vi "Main.vi"(10 "COM port name":refnum<visa-resource-name>, 11 "Module Admin":refnum<class "Delacor_lib_QMH_Cloneable Module Admin.lvclass">) -> ()   [LabVIEW 2018, in "CE14_v2.lvlib"]
doc: "This template is based off of the Queued Message Handler design pattern and the Queued Message Handler project template that ships with LabVIEW.\n\nThe main difference is that the queue is private to this module and communication between modules is performed via Broadcast and Request events.\n\nRequest events are wrapped in public API methods and are handled in the Event Handling Loop (EHL) of this VI. Any module can register for Broadcast events sent by this module. The EHL generates messages based on user interface actions.\n\nThe Message Handling Loop (MHL) processes messages generated by the EHL, or by other messages. The messages are string values, so new messages can be added easily to the Message Cases case structure in the MHL. Each message cluster can also provide an optional value for Message Data, which is a variant that can be converted to whatever message-specific data is required.\n_____\nBased on DQMH Project Template 6.0.0.91."
uses:
  CE14_v2.lvlib
  <vilib>/Delacor/Delacor QMH/Libraries/Cloneable Module Admin_class/Delacor_lib_QMH_Cloneable Module Admin.lvclass
  C:/Program Files (x86)/National Instruments/LabVIEW 2018/vi.lib/Delacor/Delacor QMH/Libraries/Module Admin_class/Delacor_lib_QMH_Module Admin.lvclass
  <vilib>/Delacor/Delacor QMH/Libraries/Message Queue_class/Delacor_lib_QMH_Message Queue.lvclass/Delacor_lib_QMH_Message Queue.ctl
  Module Data--cluster.ctl
  <vilib>/Delacor/Delacor QMH/Libraries/Cloneable Module Admin_class/Delacor_lib_QMH_Cloneable Module Admin.lvclass/Delacor_lib_QMH_Cloneable Module Admin.ctl
  Stop Argument--cluster.ctl
  <vilib>/Delacor/Delacor QMH/Libraries/Module Admin_class/Delacor_lib_QMH_Module Admin.lvclass/Delacor_lib_QMH_Module Admin.ctl
  CE14.CheckConnected Argument--cluster.ctl
  CE14.CheckConnected (Reply Payload)--cluster.ctl
  Read AC parameters Argument--cluster.ctl
  Connect to CE14 Argument--cluster.ctl
  <vilib>/Utility/miscctls.llb/LVPointTypeDef.ctl
  <vilib>/Delacor/Delacor QMH/Libraries/Message Queue_class/Delacor_lib_QMH_Enqueue Message (Single).vi
  <vilib>/Delacor/Delacor QMH/Libraries/Cloneable Module Admin_class/Delacor_lib_QMH_Get Module ID.vi
  <vilib>/Delacor/Delacor QMH/Libraries/Module Admin_class/Delacor_lib_QMH_Get External Launch.vi
  <vilib>/Utility/error.llb/Error Cluster From Error Code.vi
  <vilib>/ErrorRing/Error Ring.xnode
  <vilib>/Delacor/Delacor QMH/Libraries/Message Queue_class/Delacor_lib_QMH_Message Queue.lvclass
  Instrument Drivers/LVdriver_CE14(eMIC)/CE14_eMIC.lvlib
panel:
  out "Frequency":dbl
  out "connected":bool
  out "error out":errorcluster
  out "Status":string
  in  "Simulate EHL Error":bool
  in  "Simulate MHL Error":bool
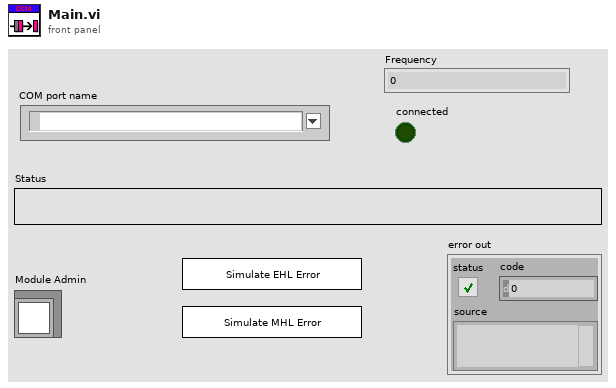
[diagram p1: front panel]
types:
  T1 = typedef "CE14_v2.lvlib/Request Events--cluster.ctl" = cluster{"Stop Module":refnum<user-event>, "Show Panel":refnum<user-event>, "Hide Panel":refnum<user-event>, "Show Diagram":refnum<user-event>, "Get Module Execution Status":refnum<user-event>, "CE14.CheckConnected":refnum<user-event>, "Read AC parameters":refnum<user-event>, "Connect to CE14":refnum<user-event>, "Stop helper loop":refnum<user-event>, "Start Helper Loop":refnum<user-event>}
  T2 = typedef "CE14_v2.lvlib/Module Data--cluster.ctl" = cluster{"Status":string, "VISA resource name":refnum<visa-resource-name>, "connected":bool}
  T3 = enum32{"invalid lock state", "Not Locked", "Locked (No Password)", "Password-protected"}
  T4 = typedef "CE14_v2.lvlib/Stop Argument--cluster.ctl" = cluster{"Module ID":i32, "Origin":string, "Exit via Stop Module Req?":bool, "Wait for Module to stop?":bool}
  T5 = typedef "CE14_v2.lvlib/CE14.CheckConnected Argument--cluster.ctl" = cluster{"Module ID":i32, "Wait Notifier":refnum<notifier>, "wait for reply":bool}
  T6 = typedef "CE14_v2.lvlib/Read AC parameters Argument--cluster.ctl" = cluster{"Module ID":i32, "Boolean":bool}
  T7 = typedef "CE14_v2.lvlib/Connect to CE14 Argument--cluster.ctl" = cluster{"Module ID":i32, "Boolean":bool}
  T8 = typedef "LVPointTypeDef.ctl" = cluster{"Horizontal":i16, "Vertical":i16}
  T9 = enum32{"Invalid", "Standard", "Closed", "Hidden", "Minimized", "Maximized"}
  T10 = typedef "CE14_v2.lvlib/CE14.CheckConnected (Reply Payload)--cluster.ctl" = cluster{"Success":bool, "CE14.CheckConnected_error":errorcluster}
  T11 = typedef "CE14_eMIC.lvlib/CE14.data.ctl" = cluster{"string":string, "float":dbl, "Name":string}
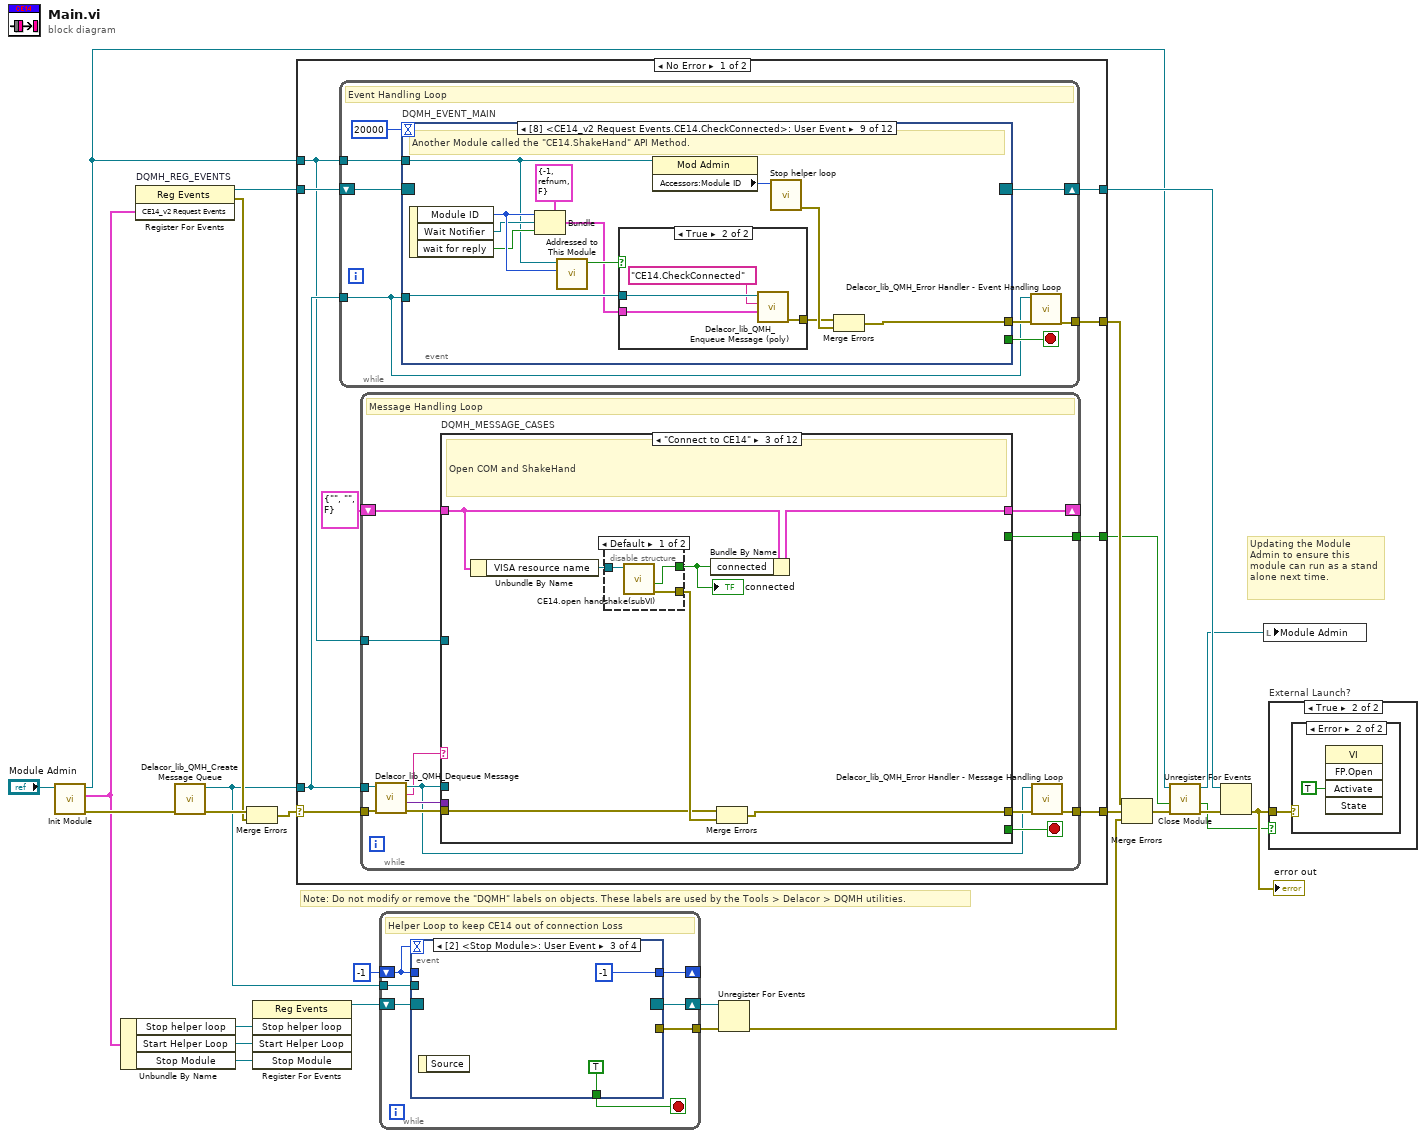
[diagram p0: block diagram]
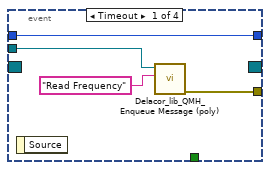
[diagram p2: hidden frame]
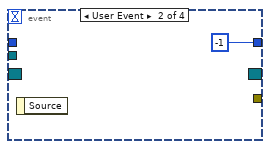
[diagram p3: hidden frame]
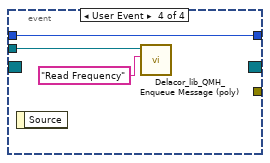
[diagram p4: hidden frame]
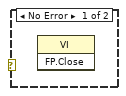
[diagram p6: hidden frame]
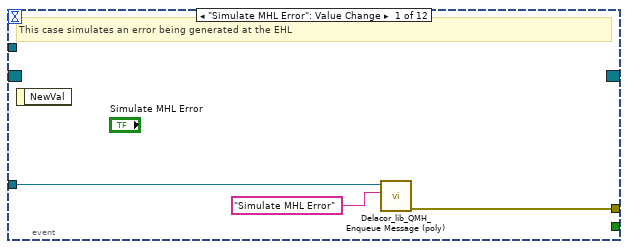
[diagram p7: hidden frame]
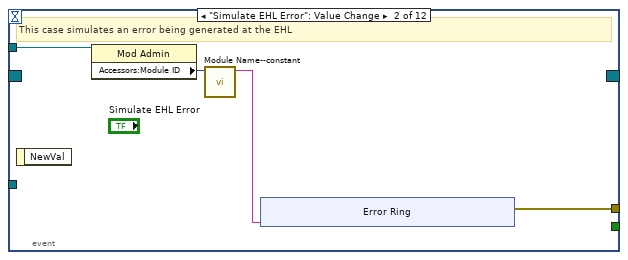
[diagram p8: hidden frame]
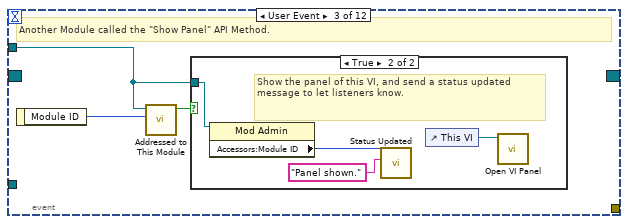
[diagram p9: hidden frame]
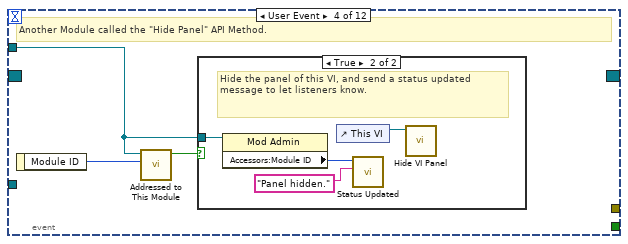
[diagram p11: hidden frame]
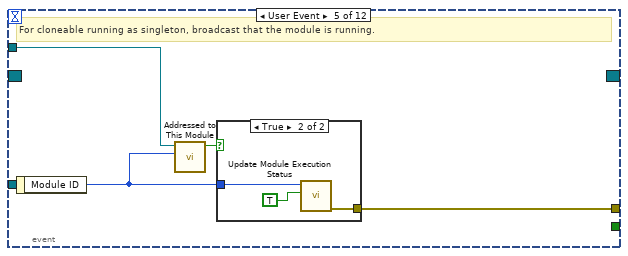
[diagram p13: hidden frame]
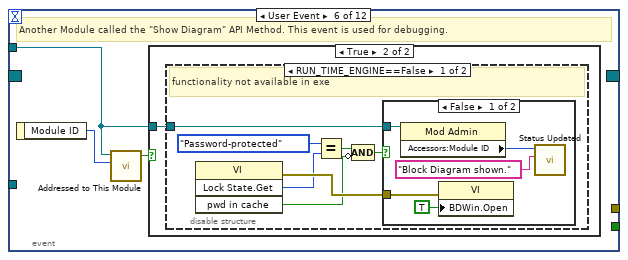
[diagram p15: hidden frame]
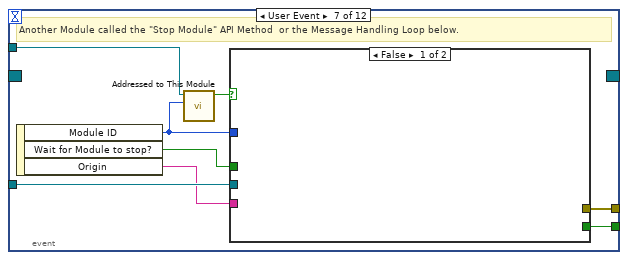
[diagram p19: hidden frame]
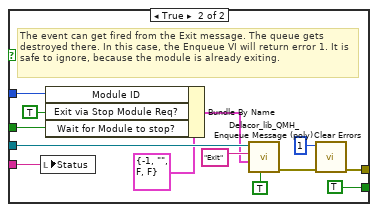
[diagram p20: hidden frame]
diagram:
  # "Note: Do not modify or remove the \"DQMH\" labels on objects. These labels are used by the Tools > Delacor > DQMH utilities."
  # "Updating the Module Admin to ensure this module can run as a stand alone next time."
  n1 = call "Init Module.vi"("Cloneable Module Admin in"="Module Admin") -> ("error out"=w23:errorcluster, "CE14_v2 Request Events"=w9:T1, "Cloneable Module Admin out"=w15:refnum<class "Delacor_lib_QMH_Cloneable Module Admin.lvclass">)  [unwired: 8 in]
  n2 = Unbundle By Name(w9) -> ("Stop helper loop"=w6:refnum<user-event>, "Start Helper Loop"=w5:refnum<user-event>, "Stop Module"=w4:refnum<user-event>)
  n3 = register-events "DQMH_REG_EVENTS"(w9) -> (reference out=w11:refnum<event-registration>, error out=w18:errorcluster)  [unwired: 2 in]
  n4 = call <vilib>:"Delacor_lib_QMH_Create Message Queue.vi"("error in"=w23) -> ("error out"=w20:errorcluster, "Message Queue"=w10:refnum<class "Delacor_lib_QMH_Message Queue.lvclass">)  [unwired: 9 in]
  n5 = Merge Errors(w20, w18) -> (w19:errorcluster)
  n6 = register-events(w6, w5, w4) -> (reference out=w8:refnum<event-registration>)  [unwired: 2 in, 1 out]
  n7 = case shown="No Error" w19 {
    selector: w19 -> [w33 w349]
    tunnel: [w35 w348] -> w24
    tunnel: [w32 w356] -> w17
    tunnel: w11 -> [w30 w356]
    tunnel: w10 -> [w29 w347]
    tunnel: [w34 _] -> w25
    tunnel: w15 -> [w28 w352]
    tunnel: [w27 _] -> w13
    frame No Error {
      n8 = while {
        tunnel: w29 -> [w37]
        shift-right: [w40] -> w32
        shift-left: w30 -> [w41]
        tunnel: [w42] -> w34
        tunnel: w28 -> [w38]
        stop <- w39 stop-if-true
        # "Event Handling Loop"
        n9 = event "DQMH_EVENT_MAIN" shown="[8] <CE14_v2 Request Events.CE14.CheckConnected>: User Event" {
          selector: w41 -> [_ _ _ _ _ _ _ _ _ _ _ _]
          dyn-events: [_ _ _ _ _ _ _ _ _ _ _ _] -> w40
          timeout: 20000 -> [_ _ _ _ _ _ _ _ _ _ _ _]
          tunnel: [_ _ _ _ _ _ w99 _ _ _ _ _] -> w39
          tunnel: w37 -> [w45 _ _ _ _ _ w101 w117 w137 w152 w167 _]
          tunnel: [w46 w50 _ _ w75 _ w102 w120 w127 w142 w158 _] -> w43
          tunnel: w38 -> [_ w49 w58 w65 w73 w79 w95 w118 w126 w145 w159 w172]
          event "Simulate MHL Error": Value Change {
            # "This case simulates an error being generated at the EHL"
            n10 = event-data() -> ()  [unwired: 1 in, 1 out]
            n11 = call-poly <vilib>:"Delacor_lib_QMH_Enqueue Message (poly).vi"("Message"="Simulate MHL Error", "Message Queue in"=w45) -> ("error out"=w46:errorcluster)  [unwired: 8 in, 1 out]
          }
          event "Simulate EHL Error": Value Change {
            # "This case simulates an error being generated at the EHL"
            n12 = event-data() -> ()  [unwired: 1 in, 1 out]
            n13 = property class="Mod Admin"(reference=w49) -> ("Accessors:Module ID"=w48:i32)  [unwired: 1 in, 2 out]
            n14 = call "Module Name--constant.vi"("Module ID"=w48) -> ("Module Name"=w47:string)  [unwired: 10 in]
            n15 = xnode "Error Ring"("parameter 0"=w47) -> ("error out"=w50:errorcluster)
          }
          event User Event {
            # "Another Module called the \"Show Panel\" API Method."
            n16 = event-data() -> ("Module ID"=w59:i32)  [unwired: 1 in]
            n17 = call "Addressed to This Module.vi"("Module ID from Argument"=w59, "Module Admin"=w58) -> ("Addressed to this instance?"=w60:bool)  [unwired: 8 in, 1 out]
            n18 = case shown="True" w60 {
              tunnel: w58 -> [_ w62]
              frame False {
              }
              frame True {
                # "Show the panel of this VI, and send a status updated message to let listeners know."
                n19 = property class="Mod Admin"(reference=w62) -> ("Accessors:Module ID"=w61:i32)  [unwired: 1 in, 2 out]
                n20 = call "Status Updated.vi"("Status"="Panel shown." ("format string"), "Module ID"=w61) -> ()  [unwired: 9 in, 1 out]
                n21 = control-ref of="This VI"() -> (w64:refnum<vi>)
                n22 = call "Open VI Panel.vi"("VI"=w64) -> ()  [unwired: 10 in, 1 out]
              }
            }
          }
          event User Event {
            # "Another Module called the \"Hide Panel\" API Method."
            n23 = event-data() -> ("Module ID"=w66:i32)  [unwired: 1 in]
            n24 = call "Addressed to This Module.vi"("Module ID from Argument"=w66, "Module Admin"=w65) -> ("Addressed to this instance?"=w67:bool)  [unwired: 8 in, 1 out]
            n25 = case shown="True" w67 {
              tunnel: w65 -> [_ w69]
              frame False {
              }
              frame True {
                # "Hide the panel of this VI, and send a status updated message to let listeners know."
                n26 = property class="Mod Admin"(reference=w69) -> ("Accessors:Module ID"=w68:i32)  [unwired: 1 in, 2 out]
                n27 = control-ref of="This VI"() -> (w71:refnum<vi>)
                n28 = call "Status Updated.vi"("Status"="Panel hidden." ("format string"), "Module ID"=w68) -> ()  [unwired: 9 in, 1 out]
                n29 = call "Hide VI Panel.vi"("VI"=w71) -> ()  [unwired: 10 in, 1 out]
              }
            }
          }
          event User Event {
            # "For cloneable running as singleton, broadcast that the module is running."
            n30 = event-data() -> ("Module ID"=w72:i32)  [unwired: 1 in]
            n31 = call "Addressed to This Module.vi"("Module ID from Argument"=w72, "Module Admin"=w73) -> ("Addressed to this instance?"=w74:bool)  [unwired: 8 in, 1 out]
            n32 = case shown="True" w74 {
              tunnel: [_ w78] -> w75
              tunnel: w72 -> [_ w77]
              frame False {
              }
              frame True {
                n33 = call "Update Module Execution Status.vi"("Running?"=TRUE, "Module ID"=w77) -> ("error out"=w78:errorcluster)  [unwired: 9 in]
              }
            }
          }
          event User Event {
            # "Another Module called the \"Show Diagram\" API Method. This event is used for debugging."
            n34 = event-data() -> ("Module ID"=w80:i32)  [unwired: 1 in]
            n35 = call "Addressed to This Module.vi"("Module ID from Argument"=w80, "Module Admin"=w79) -> ("Addressed to this instance?"=w81:bool)  [unwired: 8 in, 1 out]
            n36 = case shown="True" w81 {
              tunnel: w79 -> [_ w82]
              frame False {
              }
              frame True {
                n37 = disable-structure shown="RUN_TIME_ENGINE==False" {
                  disable-tunnel: w82 -> [w83 _]
                  frame condition #0 (active) {
                    # "functionality not available in exe"
                    n38 = invoke class="VI" method="Lock State.Get"() -> (error out=w89:errorcluster, "Get Lock State"=w88:T3, "pwd in cache"=w85:bool)  [unwired: 4 in, 1 out]
                    n39 = Equal?(x=T3."Password-protected", y=w88) -> (x = y?=w86:bool)
                    n40 = Compound Arithmetic op=AND(w86, invert w85) -> (w84:bool)
                    n41 = case shown="False" w84 {
                      tunnel: w89 -> [w94 _]
                      tunnel: w83 -> [w91 _]
                      frame False {
                        n42 = property class="Mod Admin"(reference=w91) -> ("Accessors:Module ID"=w90:i32)  [unwired: 1 in, 2 out]
                        n43 = property class="VI"(error in=w94, "BDWin.Open"=TRUE ("Block Diagram Window:Open")) -> ()  [unwired: 1 in, 2 out]
                        n44 = call "Status Updated.vi"("Status"="Block Diagram shown." ("format string"), "Module ID"=w90) -> ()  [unwired: 9 in, 1 out]
                      }
                      frame True {
                        # "Password-protected VI, and the password is not in the cache. Do not show the diagram."
                      }
                    }
                  }
                  frame condition #1 {
                  }
                }
              }
            }
          }
          event User Event {
            # "Another Module called the \"Stop Module\" API Method  or the Message Handling Loop below."
            n45 = event-data() -> ("Module ID"=w96:i32, "Wait for Module to stop?"=w98:bool, "Origin"=w97:string)  [unwired: 1 in]
            n46 = call "Addressed to This Module.vi"("Module ID from Argument"=w96, "Module Admin"=w95) -> ("Addressed to this instance?"=w100:bool)  [unwired: 8 in, 1 out]
            n47 = case shown="False" w100 {
              tunnel: [_ w114] -> w102
              tunnel: w101 -> [_ w110]
              tunnel: [_ TRUE] -> w99
              tunnel: w98 -> [_ w105]
              tunnel: w96 -> [_ w107]
              tunnel: w97 -> [_ w103]
              frame False {
              }
              frame True {
                # "The event can get fired from the Exit message. The queue gets destroyed there. In this case, the Enqueue VI will return error 1. It is safe to ignore, because the module is already exiting."
                n48 = local write "Status"(w103) -> ()
                n49 = Bundle By Name(cluster=T4 {"Module ID"=-1, "Origin"="", "Exit via Stop Module Req?"=FALSE, "Wait for Module to stop?"=FALSE} ("Stop Argument"), "Module ID"=w107, "Exit via Stop Module Req?"=TRUE, "Wait for Module to stop?"=w105) -> (w104:T4)
                n50 = call-poly <vilib>:"Delacor_lib_QMH_Enqueue Message (poly).vi"("Priority Message? (F)"=TRUE, "Message Data"=w104, "Message"="Exit", "Message Queue in"=w110) -> ("error out"=w115:errorcluster)  [unwired: 6 in, 1 out]
                n51 = call <vilib>:"Clear Errors.vi"("error in (no error)"=w115, "specific error code to clear (0: all)"=1) -> ("error out"=w114:errorcluster)  [unwired: 4 in, 1 out]
              }
            }
          }
          event Panel Close? {
            w119 = TRUE  # Discard the event, the MHL is responsible for closing and stopping this VI.
            # "Hide the panel or send the 'Exit' message if the user clicks the 'X' on the module main VI panel."
            n52 = event-data() -> ()  [unwired: 1 in, 1 out]
            n53 = property class="Mod Admin"(reference=w118) -> ("Accessors:External Launch"=w116:bool)  [unwired: 1 in, 2 out]
            n54 = case shown="False" w116 {
              tunnel: w117 -> [_ w124]
              tunnel: [_ w125] -> w120
              frame True {
                # "If externally launched, clicking the 'X' hides the panel, but doesn't close it."
                n55 = control-ref of="This VI"() -> (w121:refnum<vi>)
                n56 = call "Hide VI Panel.vi"("VI"=w121) -> ()  [unwired: 10 in, 1 out]
              }
              frame False {
                # "If run as a stand-alone VI, clicking the panel 'X' stops the VI."
                n57 = call-poly <vilib>:"Delacor_lib_QMH_Enqueue Message (poly).vi"("Priority Message? (F)"=TRUE, "Message"="Exit", "Message Queue in"=w124) -> ("error out"=w125:errorcluster)  [unwired: 7 in, 1 out]
              }
            }
            n58 = event-data("Discard?"=w119) -> ()  [unwired: 1 in, 1 out]
          }
          event User Event {
            # "Another Module called the \"CE14.ShakeHand\" API Method."
            n59 = event-data() -> ("Module ID"=w133:i32, "Wait Notifier"=w132:refnum<notifier>, "wait for reply"=w131:bool)  [unwired: 1 in]
            n60 = Bundle(cluster=T5 {"Module ID"=-1, "Wait Notifier"=refnum, "wait for reply"=FALSE} ("CE14.ShakeHand Argument"), "Module ID"=w133, "Wait Notifier"=w132, "wait for reply"=w131) -> (w134:T5)
            n61 = call "Addressed to This Module.vi"("Module ID from Argument"=w133, "Module Admin"=w126) -> ("Addressed to this instance?"=w136:bool)  [unwired: 8 in, 1 out]
            n62 = case shown="True" w136 {
              tunnel: w137 -> [_ w141]
              tunnel: w134 -> [_ w139]
              tunnel: [_ w138] -> w128
              frame False {
              }
              frame True {
                n63 = call-poly <vilib>:"Delacor_lib_QMH_Enqueue Message (poly).vi"("Message Data"=w139, "Message"="CE14.CheckConnected", "Message Queue in"=w141) -> ("error out"=w138:errorcluster)  [unwired: 7 in, 1 out]
              }
            }
            n64 = property class="Mod Admin"(reference=w126) -> ("Accessors:Module ID"=w130:i32)  [unwired: 1 in, 2 out]
            n65 = call "Stop helper loop.vi"("Module ID"=w130) -> ("error out"=w129:errorcluster)  [unwired: 10 in]
            n66 = Merge Errors(w128, w129) -> (w127:errorcluster)
          }
          event User Event {
            # "Another Module called the \"Read AC parameters\" API Method."
            n67 = event-data() -> ("Module ID"=w148:i32, "Boolean"=w147:bool)  [unwired: 1 in]
            n68 = Bundle(cluster=T6 {"Module ID"=-1, "Boolean"=FALSE} ("Read AC parameters Argument"), "Module ID"=w148, "Boolean"=w147) -> (w149:T6)
            n69 = call "Addressed to This Module.vi"("Module ID from Argument"=w148, "Module Admin"=w145) -> ("Addressed to this instance?"=w151:bool)  [unwired: 8 in, 1 out]
            n70 = case shown="True" w151 {
              tunnel: w152 -> [_ w156]
              tunnel: w149 -> [_ w153]
              tunnel: [_ w154] -> w143
              frame False {
              }
              frame True {
                n71 = call-poly <vilib>:"Delacor_lib_QMH_Enqueue Message (poly).vi"("Message Data"=w153, "Message"="Read AC parameters", "Message Queue in"=w156) -> ("error out"=w154:errorcluster)  [unwired: 7 in, 1 out]
              }
            }
            n72 = property class="Mod Admin"(reference=w145) -> ("Accessors:Module ID"=w146:i32)  [unwired: 1 in, 2 out]
            n73 = call "Stop helper loop.vi"("Module ID"=w146) -> ("error out"=w144:errorcluster)  [unwired: 10 in]
            n74 = Merge Errors(w143, w144) -> (w142:errorcluster)
          }
          event User Event {
            # "Another Module called the \"Connect to CE14\" API Method."
            n75 = event-data() -> ("Module ID"=w163:i32, "Boolean"=w162:bool)  [unwired: 1 in]
            n76 = Bundle(cluster=T7 {"Module ID"=-1, "Boolean"=FALSE} ("Connect to CE14 Argument"), "Module ID"=w163, "Boolean"=w162) -> (w164:T7)
            n77 = call "Addressed to This Module.vi"("Module ID from Argument"=w163, "Module Admin"=w159) -> ("Addressed to this instance?"=w166:bool)  [unwired: 8 in, 1 out]
            n78 = case shown="True" w166 {
              tunnel: w167 -> [_ w171]
              tunnel: w164 -> [_ w170]
              tunnel: [_ w169] -> w161
              frame False {
              }
              frame True {
                n79 = call-poly <vilib>:"Delacor_lib_QMH_Enqueue Message (poly).vi"("Message Data"=w170, "Message"="Connect to CE14", "Message Queue in"=w171) -> ("error out"=w169:errorcluster)  [unwired: 7 in, 1 out]
              }
            }
            n80 = property class="Mod Admin"(reference=w159) -> ("Accessors:Module ID"=w160:i32)  [unwired: 1 in, 2 out]
            n81 = call "Stop helper loop.vi"("Module ID"=w160) -> ("error out"=w157:errorcluster)  [unwired: 10 in]
            n82 = Merge Errors(w161, w157) -> (w158:errorcluster)
          }
          event Timeout {
            n83 = event-data() -> ()  [unwired: 1 in, 3 out]
            n84 = property class="Mod Admin"(reference=w172) -> ("Accessors:Module ID"=w173:i32)  [unwired: 1 in, 2 out]
            n85 = call "Start Helper Loop.vi"("Module ID"=w173) -> ()  [unwired: 10 in, 1 out]
          }
        }
        n86 = call-dynamic "Delacor_lib_QMH_Error Handler - Event Handling Loop.vi"("error in"=w43, "Message Queue in"=w37) -> ("dup error in"=w42:errorcluster)  [unwired: 8 in, 1 out]
      }
      n87 = while {
        tunnel: w29 -> [w178]
        shift-right: [w183] -> _
        shift-left: T2 {"Status"="", "VISA resource name"="", "connected"=FALSE} ("Data Cluster") -> [w184]
        tunnel: w33 -> [w179]
        tunnel: [w185] -> w35
        tunnel: w28 -> [w181]
        tunnel: [w180] -> w27
        stop <- w182 stop-if-true
        # "Message Handling Loop"
        n88 = call-dynamic "Delacor_lib_QMH_Dequeue Message.vi"("error in"=w179, "Message Queue in"=w178) -> ("error out"=w176:errorcluster, "Message Data"=w177:variant, "Message"=w174:string, "Message Queue out"=w175:refnum<class "Delacor_lib_QMH_Message Queue.lvclass">)  [unwired: 6 in]
        n89 = case "DQMH_MESSAGE_CASES" shown="\"Connect to CE14\"" w174 {
          selector: w174 -> [_ _ _ _ _ _ _ _ _ _ _ w335]
          tunnel: [w205 w209 w215 w222 w236 w268 w276 w278 w286 w302 w325 w337] -> w186
          tunnel: w184 -> [w189 w210 w213 w225 w242 w270 w277 w279 w285 w300 w316 w336]
          tunnel: [w198 w210 w214 w225 w242 w270 w277 w279 w285 w300 w316 w336] -> w183
          tunnel: [_ _ _ _ _ _ _ _ _ _ w323 _] -> w182
          tunnel: w177 -> [_ _ _ w232 w244 _ _ _ w284 _ w321 _]
          tunnel: w181 -> [w194 _ _ _ w238 _ _ _ w283 w298 w312 w333]
          tunnel: [_ _ _ _ _ _ _ _ _ _ w319 _] -> w180
          tunnel: w176 -> [_ w209 w211 w223 w235 w267 w276 w278 _ w296 _ w331]
          tunnel: w175 -> [_ _ _ _ _ _ _ _ w280 _ w314 _]
          frame "Initialize" {
            w191 = "Initial Message" ("Initial Message")
            # "Initialize - Any operation that needs to be done before the module can receive messages. Synchronize Caller Events.vi will inform Start Module.vi that the module has launched and is ready to receive messages. Module Did Init.vi will broadcast that the module initialized."
            n90 = call "Synchronize Caller Events.vi"("Module Admin"=w194) -> ("error out"=w206:errorcluster, "Module Admin out"=w193:refnum<class "Delacor_lib_QMH_Cloneable Module Admin.lvclass">)  [unwired: 9 in]
            n91 = property class="Mod Admin"(reference=w193) -> ("Accessors:Module ID"=w196:i32, "Accessors:External Launch"=w195:bool)  [unwired: 1 in, 2 out]
            n92 = property on="Pane" class="Pane"("Origin"=T8 {"Horizontal"=0, "Vertical"=0}) -> ()  [unwired: 2 in, 2 out]
            n93 = Bundle By Name(cluster=w189, "VISA resource name"="COM port name") -> (w190:T2)
            n94 = call "Module Name--constant.vi"("Module ID"=w196) -> ("Module Name"=w202:string)  [unwired: 10 in]
            n95 = property class="VI"("Front Panel.Title"=w202) -> (reference out=w204:refnum<vi>, error out=w208:errorcluster)  [unwired: 2 in]
            n96 = Select(t=T9."Hidden" ("State"), s=w195, f=T9."Standard" ("State")) -> (s? t:f=w199:T9)
            n97 = invoke class="VI" method="FP.Open"(reference=w204, error in=w208, "State"=w199) -> (reference out=w203:refnum<vi>, error out=w207:errorcluster)  [unwired: 2 in, 3 out]
            n98 = call "Module Name--constant.vi"("Module ID"=w196) -> ("Module Name"=w197:string)  [unwired: 10 in]
            n99 = Bundle By Name(cluster=w190, "Status"=w191) -> (w198:T2)
            n100 = invoke class="VI" method="FP.Center"(reference=w203, error in=w207) -> ()  [unwired: 1 in, 3 out]
            n101 = call "Module Did Init.vi"("error in (no error)"=w206, "Initialized?"=TRUE, "Origin"=w197, "Module ID"=w196) -> ("error out"=w205:errorcluster)  [unwired: 7 in]
            "Status" <- w191
          }
          frame "---Module Specific---", Default {
            # "Separator -- The following cases handle messages specific to this Module."
          }
          frame "Connect to CE14" {
            # "Open COM and ShakeHand"
            n102 = Unbundle By Name(w213) -> ("VISA resource name"=w217:refnum<visa-resource-name>)
            n103 = disable-structure shown="Default" {
              disable-tunnel: w217 -> [w220 _]
              disable-tunnel: [w219 _] -> w216
              disable-tunnel: [w218 TRUE] -> w212
              frame condition #0 (active) {
                n104 = call "CE14.open handshake(subVI).vi"("VISA resource name"=w220) -> ("error out"=w219:errorcluster, "success"=w218:bool)  [unwired: 7 in, 2 out]
              }
              frame condition #1 {
              }
            }
            "connected" <- w212
            n105 = Bundle By Name(cluster=w213, "connected"=w212) -> (w214:T2)
            n106 = Merge Errors(w211, w216) -> (w215:errorcluster)
          }
          frame "CE14.CheckConnected" {
            # "Open port and do shake hand produces"
            n107 = Unbundle By Name(w225) -> ("connected"=w224:bool)
            n108 = Variant To Data(type=T5 {"Module ID"=-1, "Wait Notifier"=refnum, "wait for reply"=FALSE} ("CE14.ShakeHand Argument"), Variant=w232) -> (data=w230:T5)  [unwired: 1 in, 1 out]
            n109 = Unbundle By Name(w230) -> ("Wait Notifier"=w229:refnum<notifier>, "wait for reply"=w228:bool)
            n110 = Bundle By Name(cluster=T10 {"Success"=FALSE, "CE14.CheckConnected_error"={"status"=FALSE, "code"=0, "source"=""}} ("CE14.ShakeHand (Reply Payload)"), "Success"=w224) -> (w227:T10)
            n111 = case shown="True" w228 {
              tunnel: w229 -> [_ w234]
              tunnel: w227 -> [_ w233]
              frame False {
              }
              frame True {
                n112 = Send Notification(notification=w233, notifier=w234) -> ()  [unwired: 1 in, 2 out]
              }
            }
            n113 = Merge Errors(w223) -> (w222:errorcluster)
          }
          frame "Read AC parameters" {
            # "Read ACV, ACI, PF, kW"
            n114 = Unbundle By Name(w242) -> ("VISA resource name"=w241:refnum<visa-resource-name>)
            n115 = Variant To Data(type=T6 {"Module ID"=-1, "Boolean"=FALSE} ("Read AC parameters Argument"), Variant=w244) -> ()  [unwired: 1 in, 2 out]
            n116 = disable-structure shown="Default" {
              disable-tunnel: w241 -> [w246 _]
              disable-tunnel: [w255 _] -> w240
              disable-tunnel: [w254 w264] -> w239
              frame condition #0 (active) {
                n117 = call "CE14. Read_kvar(subVI).vi"("VISA resource name"=w246) -> ("error out"=w248:errorcluster, "data out"=w249:T11, "VISA resource name out"=w247:refnum<visa-resource-name>)  [unwired: 7 in, 1 out]
                n118 = call "CE14. Read_Voltage(subVI).vi"("error in (no error)"=w248, "VISA resource name"=w247) -> ("error out"=w253:errorcluster, "data out"=w258:T11, "VISA resource name out"=w263:refnum<visa-resource-name>)  [unwired: 6 in, 1 out]
                n119 = call "CE14. Read_Current(subVI).vi"("error in (no error)"=w253, "VISA resource name"=w263) -> ("error out"=w252:errorcluster, "dataout"=w259:T11, "VISA resource name out"=w262:refnum<visa-resource-name>)  [unwired: 6 in, 1 out]
                n120 = call "CE14. Read_Freq(subVI).vi"("error in (no error)"=w252, "VISA resource name"=w262) -> ("error out"=w251:errorcluster, "data out"=w245:T11, "VISA resource name out"=w261:refnum<visa-resource-name>)  [unwired: 6 in, 1 out]
                n121 = call "CE14. Read_kW(subVI).vi"("error in (no error)"=w251, "VISA resource name"=w261) -> ("error out"=w250:errorcluster, "data out"=w257:T11, "VISA resource name out"=w260:refnum<visa-resource-name>)  [unwired: 6 in, 1 out]
                n122 = call "CE14. Read_PowerFactor(subVI).vi"("error in (no error)"=w250, "VISA resource name"=w260) -> ("error out"=w255:errorcluster, "data out"=w256:T11)  [unwired: 6 in, 2 out]
                n123 = Build Array(w256, w257, w245, w259, w258, w249) -> (w254:T11[])
              }
              frame condition #1 {
                n124 = call "Simulate CE14 data (SubVI).vi"() -> ("Array"=w264:T11[])  [unwired: 11 in]
              }
            }
            n125 = property class="Mod Admin"(reference=w238) -> ("Accessors:Module ID"=w237:i32)  [unwired: 1 in, 2 out]
            n126 = call "CE14 response data.vi"("Array"=w239, "Module ID"=w237) -> ()  [unwired: 9 in, 1 out]
            n127 = Merge Errors(w235, w240) -> (w236:errorcluster)
          }
          frame "Read Frequency" {
            n128 = Unbundle By Name(w270) -> ("VISA resource name"=w269:refnum<visa-resource-name>)
            n129 = disable-structure shown="Default" {
              disable-tunnel: w269 -> [w274 _]
              disable-tunnel: [w273 _] -> w266
              disable-tunnel: [w271 50.0 ("float")] -> w265
              frame condition #0 (active) {
                n130 = call "CE14. Read_Freq(subVI).vi"("VISA resource name"=w274) -> ("error out"=w273:errorcluster, "data out"=w272:T11)  [unwired: 7 in, 2 out]
                n131 = Unbundle By Name(w272) -> ("float"=w271:dbl)
              }
              frame condition #1 {
              }
            }
            "Frequency" <- w265
            n132 = Merge Errors(w267, w266) -> (w268:errorcluster)
          }
          frame "---Copy This Frame---" {
            # "Duplicate this frame when creating new messages.  Change this comment in the duplicated frame to describe this message."
          }
          frame "---Exit and Error Handling---" {
            # "Separator - the following cases handle errors and exit messages."
          }
          frame "Error" {
            # "Error - Check the error message data and respond accordingly. This message is sent by the \"Error Handler\" VIs at the end of each loop in this application."
            n133 = property class="Mod Admin"(reference=w283) -> ("Accessors:External Launch"=w282:bool, "Accessors:Module ID"=w281:i32)  [unwired: 1 in, 2 out]
            n134 = Variant To Data(type=errorcluster {"status"=FALSE, "code"=0, "source"=""} ("error constant"), Variant=w284) -> (data=w290:errorcluster, error out=w288:errorcluster)  [unwired: 1 in]
            n135 = call "Error Reported.vi"("Error"=w290, "Module ID"=w281) -> ()  [unwired: 9 in, 1 out]
            n136 = case shown="False" w282 {
              tunnel: [w295 _] -> w287
              tunnel: w290 -> [w294 _]
              tunnel: w280 -> [w291 _]
              frame False {
                # "If the module is running standalone, then pop up an error dialog and call the \"Exit\" message."
                n137 = call <vilib>:"Simple Error Handler.vi"("error in (no error)"=w294) -> ()  [unwired: 4 in, 5 out]
                n138 = call-poly <vilib>:"Delacor_lib_QMH_Enqueue Message (poly).vi"("Priority Message? (F)"=TRUE, "Message"="Exit", "Message Queue in"=w291) -> ("error out"=w295:errorcluster)  [unwired: 7 in, 1 out]
              }
              frame True {
                # "If the module was launched externally, calling the Error Reported broadcast VI is the only action performed by the \"Error\" message. The module's caller can then process the error appropriately."
              }
            }
            n139 = Merge Errors(w288, w287) -> (w286:errorcluster)
            n140 = local write "error out"(w286) -> ()
          }
          frame "Simulate MHL Error" {
            # "#DQMH_HowTo The 'Simulate MHL Error' button  illustrates how the MHL handles errors. This event is instructional in nature and can be removed."
            # "Simulate an error occurring at the MHL"
            n141 = property class="Mod Admin"(reference=w298) -> ("Accessors:Module ID"=w299:i32)  [unwired: 1 in, 2 out]
            n142 = call "Module Name--constant.vi"("Module ID"=w299) -> ("Module Name"=w297:string)  [unwired: 10 in]
            n143 = xnode "Error Ring"("parameter 0"=w297) -> ("error out"=w301:errorcluster)
            n144 = Merge Errors(w296, w301) -> (w302:errorcluster)
          }
          frame "Exit" {
            w323 = TRUE  # Stop the VI
            # "Release the message queue reference"
            # "Exit - Exit the application."
            n145 = Variant To Data(type=T4 {"Module ID"=-1, "Origin"="", "Exit via Stop Module Req?"=FALSE, "Wait for Module to stop?"=FALSE} ("Stop Argument"), Variant=w321) -> (data=w318:T4, error out=w324:errorcluster)  [unwired: 1 in]
            n146 = disable-structure shown="Default" {
              disable-tunnel: w316 -> [w330 _]
              disable-tunnel: [w328 _] -> w315
              frame condition #0 (active) {
                n147 = Unbundle By Name(w330) -> ("VISA resource name"=w329:refnum<visa-resource-name>)
                n148 = call "CE14 Close Connection (SubVI).vi"("VISA Refnum in"=w329) -> ("error out"=w328:errorcluster)  [unwired: 10 in]
              }
              frame condition #1 {
              }
            }
            n149 = call <vilib>:"Clear Errors.vi"("error in (no error)"=w324, "specific error code to clear (0: all)"=91 ("91: not all Exit messages will have an argument")) -> ("error out"=w327:errorcluster)  [unwired: 4 in, 1 out]
            n150 = call-dynamic "Delacor_lib_QMH_Release Message Queue.vi"("error in"=w327, "Message Queue"=w314) -> ("error out"=w326:errorcluster)  [unwired: 9 in]
            n151 = control-ref of="This VI"() -> (w317:refnum<vi>)
            n152 = property class="Mod Admin"(reference=w312) -> ("Accessors:Module ID"=w311:i32)  [unwired: 1 in, 2 out]
            n153 = call "Handle Exit.vi"("error in (no error)"=w315, "Stop Argument"=w318, "Module Admin in"=w312, "VI reference"=w317) -> ("error out"=w313:errorcluster, "Wait for Stop?"=w319:bool)  [unwired: 6 in]
            n154 = call "Stop helper loop.vi"("error in"=w313, "Module ID"=w311) -> ("error out"=w310:errorcluster)  [unwired: 9 in]
            n155 = Merge Errors(w326, w310) -> (w325:errorcluster)
          }
          frame "example" {
            # "'Default' case only runs if there is a message that isn't defined in any of the other cases.  Output a programming error."
            n156 = property class="Mod Admin"(reference=w333) -> ("Accessors:Module ID"=w332:i32)  [unwired: 1 in, 2 out]
            n157 = call "Module Name--constant.vi"("Module ID"=w332) -> ("Module Name"=w334:string)  [unwired: 10 in]
            n158 = xnode "Error Ring"("parameter 0"=w335, "parameter 1"=w334) -> ("error out"=w338:errorcluster)
            n159 = Merge Errors(w331, w338) -> (w337:errorcluster)
          }
        }
        n160 = call-dynamic "Delacor_lib_QMH_Error Handler - Message Handling Loop.vi"("error in"=w186, "Message Queue in"=w175) -> ("dup error in"=w185:errorcluster)  [unwired: 8 in, 1 out]
      }
    }
    frame Error {
      n161 = call "Synchronize Caller Events.vi"("Module Admin"=w352) -> ("Module Admin out"=w351:refnum<class "Delacor_lib_QMH_Cloneable Module Admin.lvclass">)  [unwired: 9 in, 1 out]
      n162 = property class="Mod Admin"(reference=w351) -> ("Accessors:Module ID"=w350:i32)  [unwired: 1 in, 2 out]
      n163 = call-dynamic "Delacor_lib_QMH_Release Message Queue.vi"("error in"=w349, "Message Queue"=w347) -> ("error out"=w348:errorcluster)  [unwired: 9 in]
      n164 = call "Module Name--constant.vi"("Module ID"=w350) -> ("Module Name"=w355:string)  [unwired: 10 in]
      n165 = Format Into String(format string="An error occurred during initialization. %s is no longer running.", w355) -> (resulting string=w353:string)  [unwired: 2 in, 1 out]
      n166 = call "Error Reported.vi"("Additional Information"=w353, "Error"=w348, "Module ID"=w350) -> ()  [unwired: 8 in, 1 out]
    }
  }
  n167 = while {
    shift-right: [w361] -> _
    shift-left: -1 -> [w362]
    tunnel: w10 -> [w360]
    shift-right: [w359] -> w7
    shift-left: w8 -> [w363]
    tunnel: [w357] -> w2
    stop <- w358 stop-if-true
    # "Helper Loop to keep CE14 out of connection Loss"
    n168 = event shown="[2] <Stop Module>: User Event" {
      selector: w363 -> [_ _ _ _]
      dyn-events: [_ _ _ _] -> w359
      timeout: w362 -> [_ _ _ _]
      tunnel: [_ _ TRUE _] -> w358
      tunnel: w362 -> [w367 _ _ w371]
      tunnel: [w367 -1 -1 w371] -> w361
      tunnel: w360 -> [w366 _ _ w372]
      tunnel: [w364 _ _ _] -> w357
      event Timeout {
        n169 = event-data() -> ()  [unwired: 1 in, 1 out]
        n170 = call-poly <vilib>:"Delacor_lib_QMH_Enqueue Message (poly).vi"("Message"="Read Frequency", "Message Queue in"=w366) -> ("error out"=w364:errorcluster)  [unwired: 8 in, 1 out]
      }
      event User Event {
        n171 = event-data() -> ()  [unwired: 1 in, 1 out]
      }
      event User Event {
        n172 = event-data() -> ()  [unwired: 1 in, 1 out]
      }
      event User Event {
        n173 = event-data() -> ()  [unwired: 1 in, 1 out]
        n174 = call-poly <vilib>:"Delacor_lib_QMH_Enqueue Message (poly).vi"("Message"="Read Frequency", "Message Queue in"=w372) -> ()  [unwired: 8 in, 2 out]
      }
    }
  }
  n175 = Unregister For Events(event registration refnum=w7, error in=w2) -> (error out=w1:errorcluster)
  n176 = Merge Errors(w25, w24, w1) -> (w26:errorcluster)
  n177 = call "Close Module.vi"("error in"=w26, "Wait for stop?"=w13, "Module Admin in"=w15) -> ("error out"=w22:errorcluster, "External Launch"=w12:bool, "Module Admin out"=w14:refnum<class "Delacor_lib_QMH_Cloneable Module Admin.lvclass">)  [unwired: 6 in]
  n178 = Unregister For Events(event registration refnum=w17, error in=w22) -> (error out=w21:errorcluster)
  "error out" <- w21
  n179 = local write "Module Admin"(w14) -> ()
  n180 = case "External Launch?" shown="True" w12 {
    tunnel: w21 -> [_ w374]
    frame False {
    }
    frame True {
      n181 = case shown="Error" w374 {
        frame No Error {
          n182 = invoke class="VI" method="FP.Close"() -> ()  [unwired: 3 in, 3 out]
        }
        frame Error {
          n183 = invoke class="VI" method="FP.Open"("Activate"=TRUE ("Activate?")) -> ()  [unwired: 4 in, 5 out]
        }
      }
    }
  }
